vi "Remove Icon Editor Settings.vi"(8 "error in":errorcluster) -> (0 "error out":errorcluster)   [LabVIEW 2021, in "INI Settings.lvclass"]
doc: "Clears all Icon Editor keys from the LabVIEW.ini file except for those related to the Window Position."
uses:
  INI Settings.lvclass
  INI Settings.lvclass/INI Settings.ctl
  <vilib>/Utility/config.llb/NI_LVConfig.lvlib
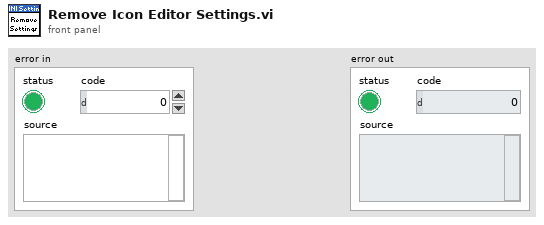
[diagram p1: front panel]
types:
  T1 = typedef "NI_LVConfig.lvlib/Config Data RefNum.ctl" = refnum<k1>
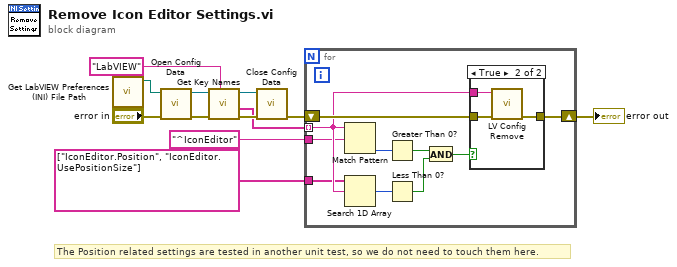
[diagram p0: block diagram]
diagram:
  # "The Position related settings are tested in another unit test, so we do not need to touch them here."
  n1 = call <resource>:"Get LabVIEW Preferences (INI) File Path.vi"() -> ("LabVIEW Preferences (INI) File Path"=w7:path)  [unwired: 11 in]
  n2 = call <vilib>:"Open Config Data.vi"("error in (no error)"="error in", "configuration file path"=w7) -> ("error out"=w12:errorcluster, "refnum"=w6:T1)  [unwired: 7 in, 1 out]
  n3 = call <vilib>:"Get Key Names.vi"("section"="LabVIEW", "error in (no error)"=w12, "refnum"=w6) -> ("error out"=w10:errorcluster, "key names"=w5:string[], "refnum out"=w1:T1)  [unwired: 5 in, 1 out]
  n4 = call <vilib>:"Close Config Data.vi"("error in (no error)"=w10, "refnum"=w1) -> ("error out"=w9:errorcluster)  [unwired: 8 in, 1 out]
  n5 = for {
    shift-right: [w21] -> w8
    shift-left: w9 -> [w22]
    tunnel: w5 -> [w20] mode=indexing
    tunnel: "^IconEditor" ("regular expression") -> [w16]
    tunnel: string[] ["IconEditor.Position", "IconEditor.UsePositionSize"] -> [w15]
    n6 = Match Pattern(string=w20, regular expression=w16) -> (offset past match=w19:i32)  [unwired: 1 in, 3 out]
    n7 = Search 1D Array(1D array=w15, element=w20) -> (index of element=w14:i32)  [unwired: 1 in]
    n8 = Greater Than 0?(x=w19) -> (x > 0?=w18:bool)
    n9 = Less Than 0?(x=w14) -> (x < 0?=w13:bool)
    n10 = And(x=w18, y=w13) -> (x .and. y?=w17:bool)
    n11 = case shown="True" w17 {
      tunnel: w22 -> [w23 w26]
      tunnel: [w23 w25] -> w21
      tunnel: w20 -> [_ w24]
      frame False {
      }
      frame True {
        n12 = call <resource>:"LV Config Remove.vi"("error in"=w26, "key"=w24) -> ("error out"=w25:errorcluster)  [unwired: 5 in]
      }
    }
  }
  "error out" <- w8
